vi "_Parse SEM Extreme Limit Check Result.vi"(8 "error in (no error)":errorcluster, 10 "Input String":string, 11 "VISA resource name":refnum<visa-resource-name>) -> (0 "error out":errorcluster, 1 "SEM Extreme Limit Check Results":T1, 2 "Reliability":i32, 3 "VISA resource name out":refnum<visa-resource-name>, 5 "Out Of Tolerance":i32)   [LabVIEW 2020, in "Rohde&Schwarz CMWXP NR FR1 Measurement.lvlib"]
uses:
  <instrlib>/Rohde&Schwarz CMWXP NR FR1 Measurement/Rohde&Schwarz CMWXP NR FR1 Measurement.lvlib
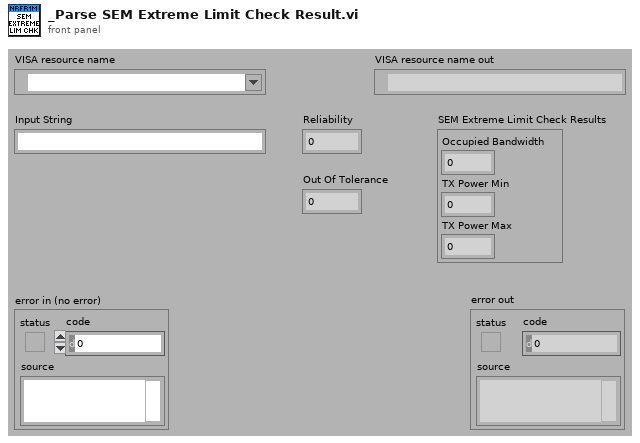
[diagram p1: front panel]
types:
  T1 = cluster{"Occupied Bandwidth":i32, "TX Power Min":i32, "TX Power Max":i32}
  T2 = cluster{"Limit Check Value":i32, "Limit Check Value":i32, "Limit Check Value":i32}
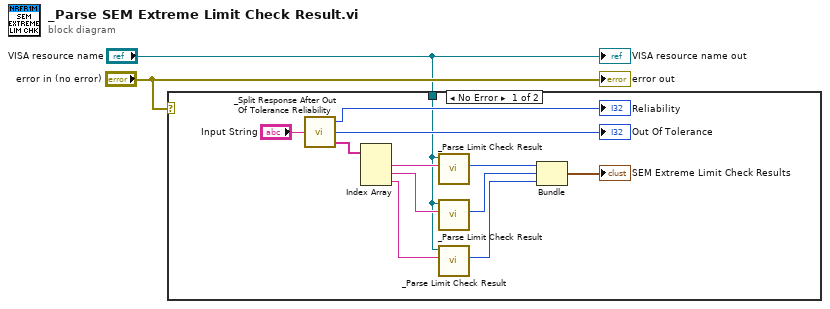
[diagram p0: block diagram]
diagram:
  n1 = case shown="No Error" "error in (no error)" {
    tunnel: "VISA resource name" -> [w3 _]
    frame No Error {
      n2 = call <instrlib>:"_Split Response After Out Of Tolerance Reliability.vi"("Input String"="Input String") -> ("Reliability out"=→"Reliability":i32, "Out Of Tolerance"=→"Out Of Tolerance":i32, "Response out"=w10:string[])
      n3 = Index Array(array=w10) -> (element #1=w9:string, element #2=w8:string, element #3=w7:string)  [unwired: 3 in]
      n4 = call <instrlib>:"_Parse Limit Check Result.vi"("String Value In"=w9, "VISA resource name"=w3) -> ("Limit Check Value"=w14:i32)  [unwired: 7 in, 2 out]
      n5 = call <instrlib>:"_Parse Limit Check Result.vi"("String Value In"=w8, "VISA resource name"=w3) -> ("Limit Check Value"=w13:i32)  [unwired: 7 in, 2 out]
      n6 = call <instrlib>:"_Parse Limit Check Result.vi"("String Value In"=w7, "VISA resource name"=w3) -> ("Limit Check Value"=w6:i32)  [unwired: 7 in, 2 out]
      n7 = Bundle("Limit Check Value"=w14, "Limit Check Value"=w13, "Limit Check Value"=w6) -> (→"SEM Extreme Limit Check Results":T2)  [unwired: 1 in]
    }
    frame Error {
    }
  }
  "error out" <- "error in (no error)"
  "VISA resource name out" <- "VISA resource name"
